vi "project.vi"() -> ()   [LabVIEW 2024]
uses:
  <vilib>/httpClient/POSTBuffer.vi
  <vilib>/Instr/_visa.llb/VISA Configure Serial Port (Instr).vi
  <vilib>/regexp/Match Regular Expression.xnode
  <vilib>/httpClient/LabVIEWHTTPClient.lvlib
panel:
  out "Data si ora pentru grafic":timestamp[](array[timestamp])
  out "valuesictdbl":dbl[](array[numeric])
  out "valuestempdbl":dbl[](array[numeric])
  out "valueshumdbl":dbl[](array[numeric])
  out "valuesict":string[](array[string])
  out "valuestemp":string[](array[string])
  out "valueshum":string[](array[string])
  out "indice comfort termic chart":dbl[](array[numeric])
  out "times":string[](array[string])
  out "valuesppmdbl":dbl[](array[numeric])
  out "valuesppm":string[](array[string])
  out "Temperatura chart":dbl[](array[numeric])
  out "Umiditate chart":dbl[](array[numeric])
  out "ppm chart":dbl[](array[numeric])
  in  "Tab Control":enum32{"Grafice realtime", "Istoric", "Setari"}(tab)
  out "Indice confort termic":dbl(knob) scale=0.0..100.0
  out "Temperatura":dbl(slide) scale=-100.0..100.0 scale format="%#_3g"
  out "Chart":dbl[](graph)
  in  "Stop":bool
  in  "Slide":i32(slide) scale=0.0..3.0
  in  "Perioada salvare in fisier":u32=1
  in  "Perioada de masurare":u32=1
  out "R0":dbl
  out "RS":dbl
  out "Umiditate":dbl
  out "Nivel CO in aer":dbl
  out "Umiditate":dbl(knob) scale=0.0..100.0
  out "Indice comfort termic":dbl
  in  "String":string
  in  "OK Button":bool
  in  "Parametru":u16(ring) items=["PPM", "Umiditate", "Temperatura", "Indice confort termic"]
  in  "Selectare data":string(combo)
  in  "Buton selectare dati":bool
  in  "Buton preluare date":bool
  out "XY Graph":cluster{timestamp[], dbl[]}(graph)
  out "Eroare la deschidere":errorcluster
  out "Eroare la configurare port":errorcluster
  out "Eroare la citire":errorcluster
  in  "Baud rate":u32(ring)=38400 items=["4800"=4800, "9600"=9600, "19200"=19200, "31250"=31250, "38400"=38400, "57600"=57600, "74880"=74880, "115200"=115200, "230400"=230400, "250000"=250000, "460800"=460800, "500000"=500000, "921600"=921600]
  in  "Port":refnum<visa-resource-name>="COM7"
  out "Eroare la inchidere port":errorcluster
  out "Eroare la preluarea din string":errorcluster
  out "Eroare la decodificare":errorcluster
  in  "data bits (8)":u16=8 min=5 max=8 step=1
  in  "parity (0:none)":enum16{"None", "Odd", "Even", "Mark", "Space"}(ring)
  in  "stop bits (10: 1 bit)":u16(ring)=10 items=["1.0"=10, "1.5"=15, "2.0"=20]
  in  "flow control (0:none)":u16(ring) items=["None", "XON/XOFF", "RTS/CTS", "XON/XOFF & RTS/CTS", "DTR/DSR", "XON/XOFF & DTR/DSR"]
  # "Informatii senzor gaz (Kohmi)"
  # "Perioada salvare"
  # "Setari canal"
  # "Erori"
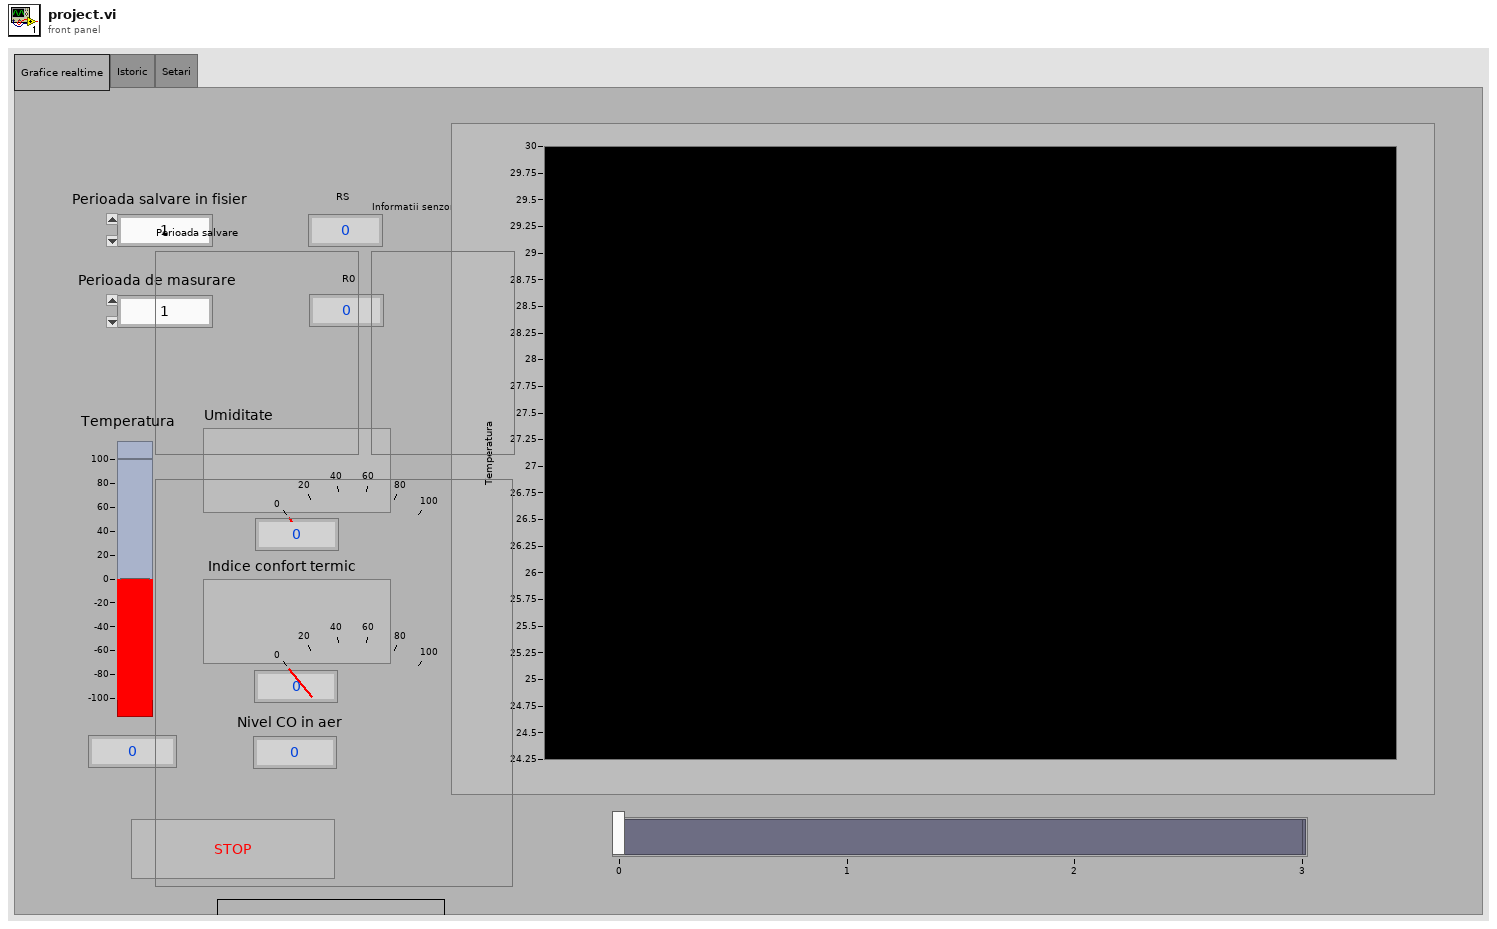
[diagram p1: front panel]
types:
  T1 = typedef "LabVIEWHTTPClient.lvlib/ClientHandle.ctl" = refnum<k1>
  T2 = cluster{"times":string[], "valuesppm":string[], "valueshum":string[], "valuestemp":string[], "valuesict":string[]}
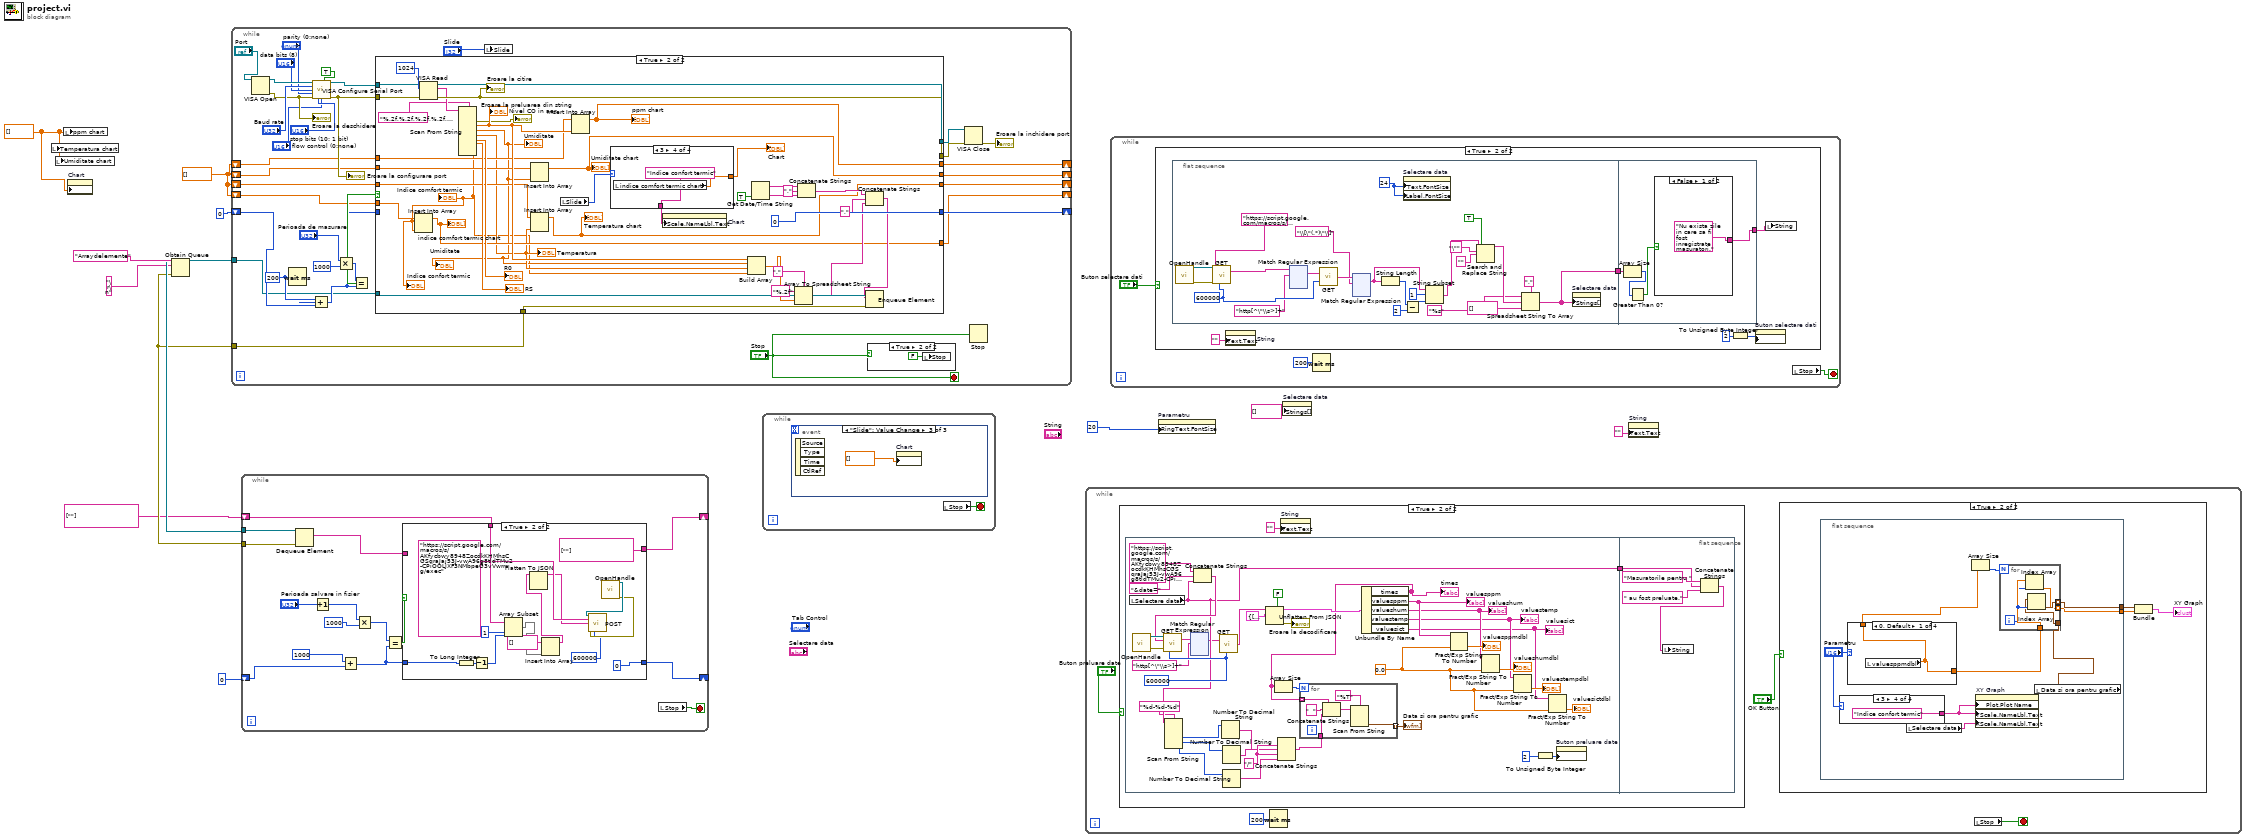
[diagram p0: block diagram]
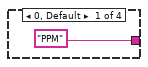
[diagram p3: hidden frame]
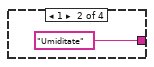
[diagram p4: hidden frame]
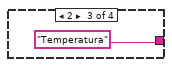
[diagram p5: hidden frame]
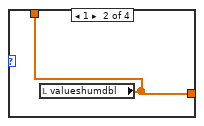
[diagram p6: hidden frame]
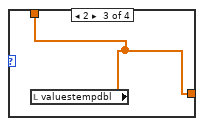
[diagram p7: hidden frame]
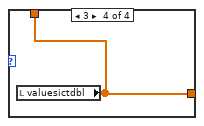
[diagram p8: hidden frame]
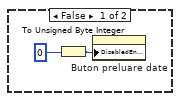
[diagram p9: hidden frame]
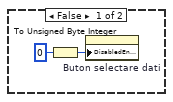
[diagram p10: hidden frame]
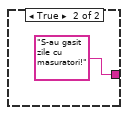
[diagram p11: hidden frame]
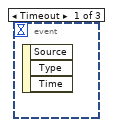
[diagram p12: hidden frame]
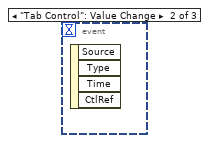
[diagram p13: hidden frame]
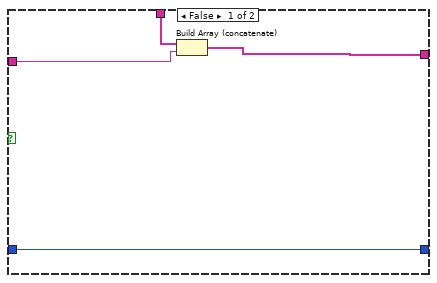
[diagram p14: hidden frame]
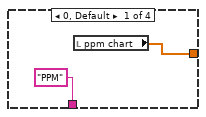
[diagram p17: hidden frame]
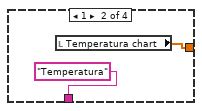
[diagram p18: hidden frame]
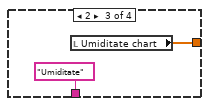
[diagram p19: hidden frame]
diagram:
  w3 = dbl[] []
  w5 = dbl[] []
  n1 = local write "Temperatura chart"(w5) -> ()
  n2 = local write "Umiditate chart"(w5) -> ()
  n3 = local write "ppm chart"(w5) -> ()
  n4 = property on="Chart" class="WFChart (strict)"("History Data"=w5) -> ()  [unwired: 2 in, 2 out]
  n5 = Obtain Queue(name (unnamed)="Arraydelemente", element data type="\r\n" ("spreadsheet string 2")) -> (queue out=w10:refnum<queue>, error out=w9:errorcluster)  [unwired: 3 in, 1 out]
  n6 = while {
    shift-right: [w40] -> _
    shift-left: u32 0 ("milliseconds to wait") -> [w45]
    tunnel: w10 -> [w35]
    tunnel: w9 -> [w34]
    shift-right: [w30] -> _
    shift-left: w3 -> [w31]
    shift-right: [w28] -> _
    shift-left: w3 -> [w29]
    shift-right: [w26] -> _
    shift-left: w3 -> [w27]
    shift-right: [w24] -> _
    shift-left: w3 -> [w25]
    stop <- "Stop" stop-if-true
    w46 = u32 200 ("milliseconds to wait")
    n7 = VISA Open(VISA resource name="Port") -> (VISA resource name=w23:refnum<visa-resource-name>, error out=w21:errorcluster)  [unwired: 4 in]
    "Eroare la deschidere" <- w21
    n8 = Wait (ms)(milliseconds to wait=w46) -> ()  [unwired: 1 out]
    n9 = call-poly "VISA Configure Serial Port"("VISA resource name"=w23, "Enable Termination\nChar (T)"=TRUE ("Enable Termination\nChar (T)"), "baud rate (9600)"="Baud rate", "data bits (8)"="data bits (8)", "parity (0:none)"="parity (0:none)", "error in (no error)"=w21, "stop bits (10: 1 bit)"="stop bits (10: 1 bit)", "flow control (0:none)"="flow control (0:none)") -> ("VISA resource name out"=w37:refnum<visa-resource-name>, "error out"=w33:errorcluster)  [unwired: 6 in]
    "Eroare la configurare port" <- w33
    n10 = Add(x=w46, y=w45) -> (x+y=w39:u32)
    n11 = Multiply(x="Perioada de masurare", y=u32 1000) -> (x*y=w41:u32)
    n12 = Equal?(x=w41, y=w39) -> (x = y?=w44:bool)
    n13 = case shown="True" w44 {
      tunnel: [w50 u32 0 ("milliseconds to wait")] -> w40
      tunnel: w39 -> [w50 _]
      tunnel: w33 -> [w48 w88]
      tunnel: w37 -> [w49 w86]
      tunnel: [w49 w85] -> w18
      tunnel: [w48 w71] -> w19
      tunnel: w35 -> [_ w82]
      tunnel: w34 -> [_ w81]
      tunnel: w31 -> [_ w66]
      tunnel: [_ w65] -> w30
      tunnel: w29 -> [_ w64]
      tunnel: [_ w63] -> w28
      tunnel: w27 -> [_ w62]
      tunnel: [_ w61] -> w26
      tunnel: w25 -> [_ w59]
      tunnel: [_ w58] -> w24
      frame False {
      }
      frame True {
        n14 = VISA Read(VISA resource name=w86, byte count=u32 1024, error in (no error)=w88) -> (VISA resource name out=w85:refnum<visa-resource-name>, read buffer=w68:string, error out=w71:errorcluster)  [unwired: 1 out]
        "Eroare la citire" <- w71
        n15 = Scan From String(format string="%.2f,%.2f,%.2f,%.2f,%.2f,%.2f,%.2f", input string=w68) -> (error out=→"Eroare la preluarea din string":errorcluster, output 1=w69:dbl, output 2=w56:dbl, output 3=w57:dbl, output 4=→"R0":dbl, output 5=→"RS":dbl, output 7=w55:dbl)  [unwired: 10 in, 2 out]
        "Nivel CO in aer" <- w69
        "Umiditate" <- w56
        "Indice comfort termic" <- w55
        "Temperatura" <- w57
        "Umiditate" <- w56
        "Indice confort termic" <- w55
        n16 = Insert Into Array(array=w59, new element=w55) -> (w58:dbl[])  [unwired: 1 in]
        "indice comfort termic chart" <- w58
        n17 = Insert Into Array(array=w64, new element=w56) -> (w63:dbl[])  [unwired: 1 in]
        "Umiditate chart" <- w63
        n18 = Insert Into Array(array=w62, new element=w57) -> (w61:dbl[])  [unwired: 1 in]
        "Temperatura chart" <- w61
        n19 = local read "Slide"() -> (w70:i32)
        n20 = Insert Into Array(array=w66, new element=w69) -> (w65:dbl[])  [unwired: 1 in]
        "ppm chart" <- w65
        n21 = case shown="3" w70 {
          tunnel: [w91 w93 w95 w97] -> w52
          tunnel: ["PPM" "Temperatura" "Umiditate" "Indice confort termic"] -> w51
          frame 0, Default {
            n22 = local read "ppm chart"() -> (w91:dbl[])
          }
          frame 1 {
            n23 = local read "Temperatura chart"() -> (w93:dbl[])
          }
          frame 2 {
            n24 = local read "Umiditate chart"() -> (w95:dbl[])
          }
          frame 3 {
            n25 = local read "indice comfort termic chart"() -> (w97:dbl[])
          }
        }
        "Chart" <- w52
        n26 = property on="Chart" class="WFChart (strict)"("YScale.NameLbl.Text"=w51) -> ()  [unwired: 2 in, 2 out]
        n27 = Build Array(w69, w56, w57, w55) -> (w80:dbl[])
        n28 = Get Date/Time String(want seconds? (F)=TRUE) -> (date string=w54:string, time string=w53:string)  [unwired: 2 in]
        n29 = Array To Spreadsheet String(delimiter (Tab)=",", array=w80, 3:"%.2f" ("format string")) -> (spreadsheet string=w74:string)
        n30 = Concatenate Strings(w54, "," ("string"), w53) -> (w75:string)
        n31 = Concatenate Strings(w75, "," ("string"), w74) -> (w72:string)
        n32 = Enqueue Element(queue=w82, element=w72, error in (no error)=w81) -> ()  [unwired: 1 in, 3 out]
      }
    }
    n33 = local write "Slide"("Slide") -> ()
    n34 = case shown="True" "Stop" {
      frame False {
      }
      frame True {
        n35 = local write "Stop"(FALSE ("stop")) -> ()
      }
    }
    n36 = VISA Close(VISA resource name=w18, error in (no error)=w19) -> (error out=→"Eroare la inchidere port":errorcluster)
    n37 = Stop(stop? (T)="Stop") -> ()
  }
  n38 = while {
    tunnel: w10 -> [w107]
    tunnel: w9 -> [w106]
    shift-right: [w104] -> _
    shift-left: u32 0 ("milliseconds to wait") -> [w103]
    shift-right: [w100] -> _
    shift-left: string[] [""] ("Array") -> [w101]
    stop <- w112 stop-if-true
    n39 = Dequeue Element(queue=w107, error in (no error)=w106) -> (element=w102:string)  [unwired: 1 in, 3 out]
    n40 = Increment(x="Perioada salvare in fisier") -> (x+1=w98:u32)
    n41 = Add(x=u32 1000 ("milliseconds to wait"), y=w103) -> (x+y=w105:u32)
    n42 = Multiply(x=w98, y=u32 1000) -> (x*y=w110:u32)
    n43 = Equal?(x=w110, y=w105) -> (x = y?=w108:bool)
    n44 = case shown="True" w108 {
      tunnel: w105 -> [w116 w127]
      tunnel: [w116 u32 0 ("milliseconds to wait")] -> w104
      tunnel: w102 -> [w115 _]
      tunnel: w101 -> [w114 w129]
      tunnel: [w113 string[] [""] ("Array")] -> w100
      frame False {
        n45 = Build Array (concatenate)(w114, w115) -> (w113:string[])
      }
      frame True {
        n46 = To Long Integer(number=w127) -> (32bit integer=w126:i32)
        n47 = Decrement(x=w126) -> (x-1=w125:i32)
        n48 = Array Subset(array=w129, index=1, length=w125) -> (w121:string[])
        n49 = Insert Into Array(array=string[] [], new element=w121) -> (w120:string[])  [unwired: 1 in]
        n50 = Flatten To JSON(anything=w120) -> (JSON string=w123:string)  [unwired: 2 in, 1 out]
        n51 = call <vilib>:"OpenHandle.vi"() -> ("client handle out"=w119:T1, "error out"=w118:errorcluster)  [unwired: 14 in]
        n52 = call-poly <vilib>:"POST.vi"("client handle"=w119, "url"="https://script.google.com/macros/s/AKfycbwy8948ZocdkKHMhsCGSqraJaj53J-vwA96g8tldTMu2-CPiOOLJXF3NMbpeG3vVwrrrg/exec", "buffer"=w123, "error in (no error)"=w118, "timeout (10000)"=600000) -> ()  [unwired: 7 in, 4 out]
      }
    }
    n53 = local read "Stop"() -> (w112:bool)
  }
  n54 = while {
    stop <- w132 stop-if-true
    n55 = event shown="[2] \"Slide\": Value Change" {
      selector: _ -> [_ _ _]
      dyn-events: _ -> [_ _ _]
      timeout: _ -> [_ _ _]
      event Timeout {
        n56 = event-data() -> ()  [unwired: 1 in, 3 out]
      }
      event "Tab Control": Value Change {
        n57 = event-data() -> ()  [unwired: 1 in, 4 out]
      }
      event "Slide": Value Change {
        n58 = event-data() -> ()  [unwired: 1 in, 4 out]
        n59 = property on="Chart" class="WFChart (strict)"("History Data"=dbl[] []) -> ()  [unwired: 2 in, 2 out]
      }
    }
    n60 = local read "Stop"() -> (w132:bool)
  }
  n61 = while {
    stop <- w137 stop-if-true
    n62 = case shown="True" "Buton preluare date" {
      frame False {
        n63 = To Unsigned Byte Integer(number=0) -> (unsigned 8bit integer=w164:u8)
        n64 = property on="Buton preluare date" class="Bool"("DisabledEnum"=w164) -> ()  [unwired: 2 in, 2 out]
      }
      frame True {
        n65 = flat-sequence {
          tunnel: [w179] -> w166
          tunnel: w166 -> [w329]
          frame #0 {
            w177 = "/" ("string")
            w194 = 600000 ("timeout (10000)")
            w189 = 0.0
            n66 = local read "Selectare data"() -> (w179:string)
            n67 = call <vilib>:"OpenHandle.vi"() -> ("client handle out"=w203:T1, "error out"=w204:errorcluster)  [unwired: 14 in]
            n68 = Scan From String(format string="%d-%d-%d", input string=w179) -> (output 1=w176:i32, output 2=w174:i32, output 3=w172:i32)  [unwired: 5 in, 3 out]
            n69 = Concatenate Strings("https://script.google.com/macros/s/AKfycbwy8948ZocdkKHMhsCGSqraJaj53J-vwA96g8tldTMu2-CPiOOLJXF3NMbpeG3vVwrrrg/exec?command=getValues" ("url"), "&date=" ("string"), w179) -> (w199:string)
            n70 = call <vilib>:"GET.vi"("client handle"=w203, "url"=w199, "error in (no error)"=w204, "timeout (10000)"=w194) -> ("headers"=w169:string)  [unwired: 8 in, 3 out]
            n71 = xnode ("Match Regular Expression")("input string"=w169, "regular expression"="http[^\"\\s>]+") -> ("whole match"=w167:string)  [unwired: 4 in, 4 out]
            n72 = call <vilib>:"GET.vi"("url"=w167, "timeout (10000)"=w194) -> ("body"=w168:string)  [unwired: 10 in, 3 out]
            n73 = Number To Decimal String(number=w176) -> (decimal integer string=w175:string)  [unwired: 1 in]
            n74 = Number To Decimal String(number=w174) -> (decimal integer string=w173:string)  [unwired: 1 in]
            n75 = Number To Decimal String(number=w172) -> (decimal integer string=w171:string)  [unwired: 1 in]
            n76 = Unflatten From JSON(enable LabVIEW extensions? (T)=FALSE, JSON string=w168, type and defaults=T2 {"times"=[], "valuesppm"=[], "valueshum"=[], "valuestemp"=[], "valuesict"=[]} ("Cluster")) -> (value=w190:T2, error out=→"Eroare la decodificare":errorcluster)  [unwired: 4 in]
            n77 = Concatenate Strings(w173, w177, w175, w177, w171) -> (w170:string)
            n78 = Unbundle By Name(w190) -> ("times"=w181:string[], "valuesppm"=w202:string[], "valueshum"=w187:string[], "valuestemp"=w186:string[], "valuesict"=w184:string[])
            "valuesppm" <- w202
            "times" <- w181
            "valueshum" <- w187
            "valuestemp" <- w186
            "valuesict" <- w184
            n79 = Array Size(array=w181) -> (size(s)=w182:i32)
            n80 = for {
              N: w182 -> [_]
              tunnel: w181 -> [w327] mode=indexing
              tunnel: [w324] -> w180 mode=indexing
              tunnel: w170 -> [w323]
              n81 = Concatenate Strings(w327, "  " ("string"), w323) -> (w322:string)
              n82 = Scan From String(format string="%T", input string=w322) -> (output 1=w324:timestamp)  [unwired: 3 in, 3 out]
            }
            "Data si ora pentru grafic" <- w180
            n83 = Fract/Exp String To Number(string=w202, default (0 dbl)=w189) -> (number=→"valuesppmdbl":dbl[])  [unwired: 2 in, 1 out]
            n84 = Fract/Exp String To Number(string=w187, default (0 dbl)=w189) -> (number=→"valueshumdbl":dbl[])  [unwired: 2 in, 1 out]
            n85 = Fract/Exp String To Number(string=w186, default (0 dbl)=w189) -> (number=→"valuestempdbl":dbl[])  [unwired: 2 in, 1 out]
            n86 = To Unsigned Byte Integer(number=2) -> (unsigned 8bit integer=w191:u8)
            n87 = Fract/Exp String To Number(string=w184, default (0 dbl)=w189) -> (number=→"valuesictdbl":dbl[])  [unwired: 2 in, 1 out]
            n88 = property on="Buton preluare date" class="Bool"("DisabledEnum"=w191) -> ()  [unwired: 2 in, 2 out]
          }
          frame #1 {
            n89 = Concatenate Strings("Masuratorile pentru ", w329, " au fost preluate.") -> (w331:string)
            n90 = local write "String"(w331) -> ()
          }
        }
        n91 = property on="String" class="Str"("Text.Text"="") -> ()  [unwired: 2 in, 2 out]
      }
    }
    n92 = Wait (ms)(milliseconds to wait=u32 200) -> ()  [unwired: 1 out]
    n93 = case shown="True" "OK Button" {
      frame False {
      }
      frame True {
        n94 = flat-sequence {
          tunnel: [w142] -> w140
          tunnel: [w141] -> w139
          frame #0 {
            n95 = case shown="3" "Parametru" {
              tunnel: ["PPM" ("Plot.Plot Name") "Umiditate" ("Plot.Plot Name") "Temperatura" ("Plot.Plot Name") "Indice confort termic" ("Plot.Plot Name")] -> w144
              frame 0, Default {
              }
              frame 1 {
              }
              frame 2 {
              }
              frame 3 {
              }
            }
            n96 = case shown="0, Default" "Parametru" {
              tunnel: [w159 w160 w161 w162] -> w148
              tunnel: [w159 w160 w161 w162] -> w147
              frame 0, Default {
                n97 = local read "valuesppmdbl"() -> (w159:dbl[])
              }
              frame 1 {
                n98 = local read "valueshumdbl"() -> (w160:dbl[])
              }
              frame 2 {
                n99 = local read "valuestempdbl"() -> (w161:dbl[])
              }
              frame 3 {
                n100 = local read "valuesictdbl"() -> (w162:dbl[])
              }
            }
            n101 = local read "Selectare data"() -> (w143:string)
            n102 = Array Size(array=w148) -> (size(s)=w146:i32)
            n103 = property on="XY Graph" class="XYGraph (strict)"("Plot.Plot Name"=w144, "YScale.NameLbl.Text"=w144, "XScale.NameLbl.Text"=w143) -> ()  [unwired: 2 in, 2 out]
            n104 = local read "Data si ora pentru grafic"() -> (w145:timestamp[])
            n105 = for {
              N: w146 -> [_]
              tunnel: [w152] -> w142 mode=indexing
              tunnel: [w151] -> w141 mode=indexing
              tunnel: w147 -> [w154]
              tunnel: w145 -> [w150]
              i -> [w153]
              n106 = Index Array(array=w154, index=w153) -> (element=w151:dbl)
              n107 = Index Array(array=w150, index=w153) -> (element=w152:timestamp)
            }
          }
        }
        n108 = Bundle(w140, w139) -> (→"XY Graph":cluster{timestamp[], dbl[]})  [unwired: 1 in]
      }
    }
    n109 = local read "Stop"() -> (w137:bool)
  }
  n110 = while {
    stop <- w333 stop-if-true
    n111 = case shown="True" "Buton selectare dati" {
      frame False {
        n112 = To Unsigned Byte Integer(number=0) -> (unsigned 8bit integer=w336:u8)
        n113 = property on="Buton selectare dati" class="Bool"("DisabledEnum"=w336) -> ()  [unwired: 2 in, 2 out]
      }
      frame True {
        n114 = flat-sequence {
          tunnel: [w342] -> w338
          tunnel: [w603] -> w339
          tunnel: w338 -> [w600]
          frame #0 {
            w345 = 600000 ("timeout (10000)")
            w352 = u32 24 ("Label.Font:Size")
            n115 = call <vilib>:"OpenHandle.vi"() -> ("client handle out"=w357:T1, "error out"=w356:errorcluster)  [unwired: 14 in]
            n116 = call <vilib>:"GET.vi"("client handle"=w357, "url"="https://script.google.com/macros/s/AKfycbwy8948ZocdkKHMhsCGSqraJaj53J-vwA96g8tldTMu2-CPiOOLJXF3NMbpeG3vVwrrrg/exec?command=getAllDates", "error in (no error)"=w356, "timeout (10000)"=w345) -> ("headers"=w364:string)  [unwired: 8 in, 3 out]
            n117 = xnode ("Match Regular Expression")("input string"=w364, "regular expression"="http[^\"\\s>]+") -> ("whole match"=w365:string)  [unwired: 4 in, 4 out]
            n118 = call <vilib>:"GET.vi"("url"=w365, "timeout (10000)"=w345) -> ("body"=w361:string)  [unwired: 10 in, 3 out]
            n119 = xnode ("Match Regular Expression")("input string"=w361, "regular expression"="\\[\"(.*)\"\\]") -> ("whole match"=w360:string)  [unwired: 4 in, 4 out]
            n120 = String Length(string=w360) -> (length=w362:i32)
            n121 = property on="Selectare data" class="CmbBox"("Text.FontSize"=w352, "Label.FontSize"=w352) -> ()  [unwired: 2 in, 2 out]
            n122 = Subtract(x=w362, y=2) -> (x-y=w363:i32)
            n123 = String Subset(string=w360, offset (0)=1, length (rest)=w363) -> (substring=w359:string)
            n124 = Search and Replace String(replace all?=TRUE ("replace all? (F)"), input string=w359, search string="\"", replace string="" ("replace string (\"\")")) -> (result string=w358:string)  [unwired: 4 in, 3 out]
            n125 = Spreadsheet String To Array(delimiter (Tab)=",", format string="%s", spreadsheet string=w358, array type (2D Dbl)=string[] []) -> (array=w342:string[])
            n126 = property on="Selectare data" class="CmbBox"("Strings[]"=w342) -> ()  [unwired: 2 in, 2 out]
          }
          frame #1 {
            n127 = Array Size(array=w600) -> (size(s)=w601:i32)
            n128 = Greater Than 0?(x=w601) -> (x > 0?=w602:bool)
            n129 = case shown="False" w602 {
              tunnel: ["Nu exista zile in care sa fi fost inregistrate masuratori." ("string") "S-au gasit zile cu masuratori!" ("string")] -> w603
              frame False {
              }
              frame True {
              }
            }
          }
        }
        n130 = property on="String" class="Str"("Text.Text"="") -> ()  [unwired: 2 in, 2 out]
        n131 = To Unsigned Byte Integer(number=2) -> (unsigned 8bit integer=w341:u8)
        n132 = property on="Buton selectare dati" class="Bool"("DisabledEnum"=w341) -> ()  [unwired: 2 in, 2 out]
        n133 = local write "String"(w339) -> ()
      }
    }
    n134 = Wait (ms)(milliseconds to wait=u32 200) -> ()  [unwired: 1 out]
    n135 = local read "Stop"() -> (w333:bool)
  }
  n136 = property on="Parametru" class="Ring (strict)"("RingText.FontSize"=u32 20 ("Ring Text.Font:Size")) -> ()  [unwired: 2 in, 2 out]
  n137 = property on="Selectare data" class="CmbBox"("Strings[]"=string[] []) -> ()  [unwired: 2 in, 2 out]
  n138 = property on="String" class="Str"("Text.Text"="") -> ()  [unwired: 2 in, 2 out]
